vi "Verify Current.vi"(8 "error in":errorcluster, 11 "6700 in":refnum<class "6700.lvclass">) -> (0 "error out":errorcluster, 3 "6700 out":refnum<class "6700.lvclass">)   [LabVIEW 2018, in "6700.lvlib" / "6700.lvclass"]
uses:
  6700.lvclass
  6700.lvclass/6700.ctl
  builds/Power_Supply.lvlibp/Power Supply.lvclass
  C:/Users/Ron.Dexter.LUMINARTECH/Desktop/builds/Power_Supply.lvlibp/Power Supply.lvclass
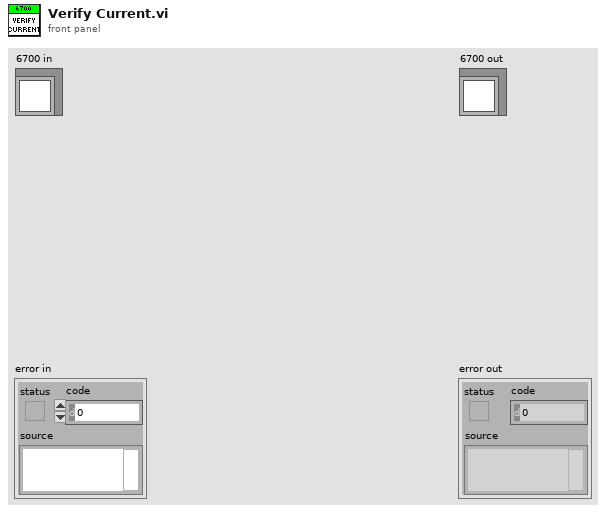
[diagram p1: front panel]
types:
  T1 = typedef "Power_Supply.lvlibp/Supply Settings.ctl" = cluster{"Voltage":dbl, "Current":dbl, "Output":bool}
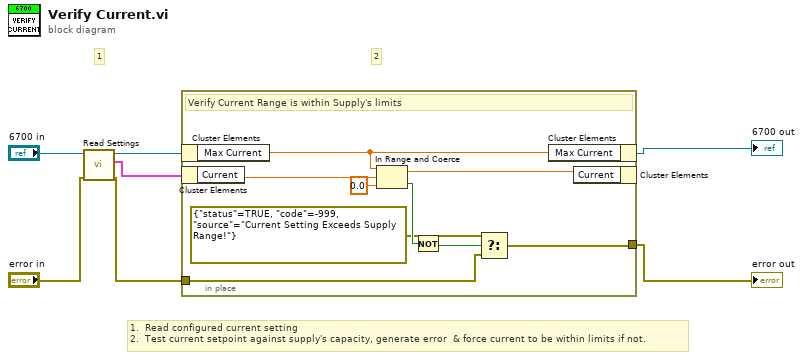
[diagram p0: block diagram]
diagram:
  # "2"
  # "1"
  # "1.  Read configured current setting\n2.  Test current setpoint against supply's capacity, generate error  & force current to be within limits if not."
  n1 = call "Read Settings.vi"("error in (no error)"="error in", "Power Supply in"="6700 in") -> ("error out"=w1:errorcluster, "Settings"=w5:T1, "Power Supply out"=w3:refnum<class "6700.lvclass">)  [unwired: 7 in]
  n2 = in-place {
    in-place-border: w1 -> [w11]
    in-place-border: [w10] -> w6
    # "Verify Current Range is within Supply's limits"
    n3 = in-place-cluster #1(w3) -> ("Max Current"=w16:dbl)
    n4 = in-place-cluster #2(w5) -> ("Current"=w15:dbl)
    n5 = In Range and Coerce(upper limit=w16, x=w15, lower limit=0.0) -> (coerced(x)=w14:dbl, In Range?=w13:bool)
    n6 = Not(x=w13) -> (.not. x?=w12:bool)
    n7 = Select(t=errorcluster {"status"=TRUE, "code"=-999, "source"="Current Setting Exceeds Supply Range!"} ("error out"), s=w12, f=w11) -> (s? t:f=w10:errorcluster)
    n8 = in-place-cluster #1("Max Current"=w16) -> (→"6700 out":refnum<class "6700.lvclass">)
    n9 = in-place-cluster #2("Current"=w14) -> ()  [unwired: 1 out]
  }
  "error out" <- w6
